vi "Pause.vi"(8 "error in":errorcluster, 9 "timeout (-1)":i32=-1, 11 "Engine Runtime Interface in":refnum<class "Engine Runtime Interface.lvclass">) -> (0 "error out":errorcluster, 3 "Engine Runtime Interface out":refnum<class "Engine Runtime Interface.lvclass">)   [LabVIEW 2014, in "Engine Runtime Interface.lvclass"]
doc: "This function pauses the execution of an engine in the running state. Once paused, the engine can continue running using the 'Start' function or be told to uninitialize using the 'Stop' function."
uses:
  Engine Runtime Interface.lvclass
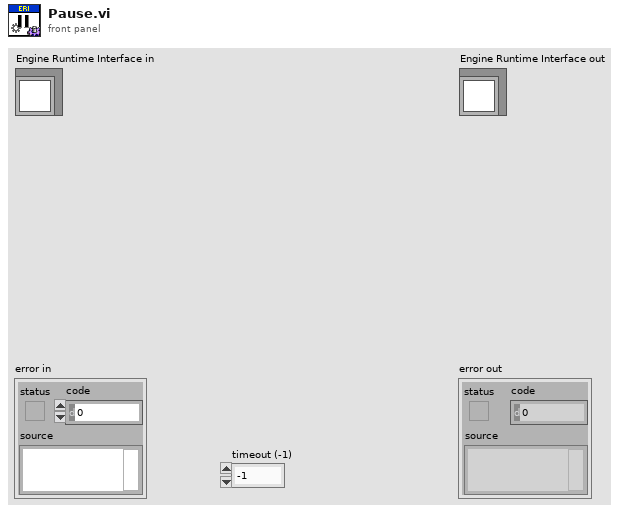
[diagram p1: front panel]
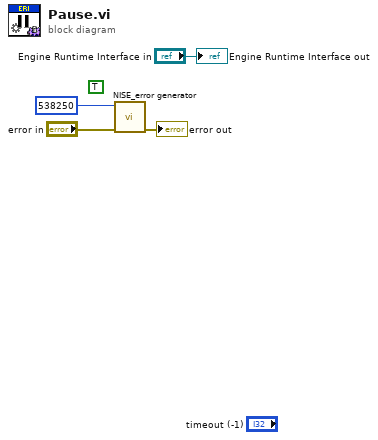
[diagram p0: block diagram]
diagram:
  (unwired) TRUE ("show call chain? (False)")
  n1 = call <vilib>:"NISE_error generator.vi"("error in"="error in", "error code (0)"=538250) -> ("error out"=→"error out":errorcluster)  [unwired: 7 in]
  "Engine Runtime Interface out" <- "Engine Runtime Interface in"
